vi "Arrays.vi"() -> ()   [LabVIEW 2018]
panel:
  out "Subset Array":dbl[][](array[numeric])
  out "Scaled Array":dbl[][](array[numeric])
  out "Random Array":dbl[][](array[numeric])
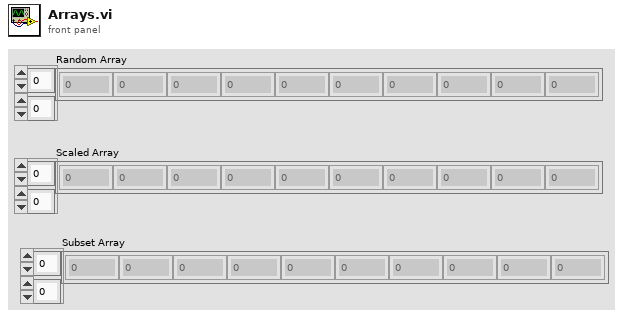
[diagram p1: front panel]
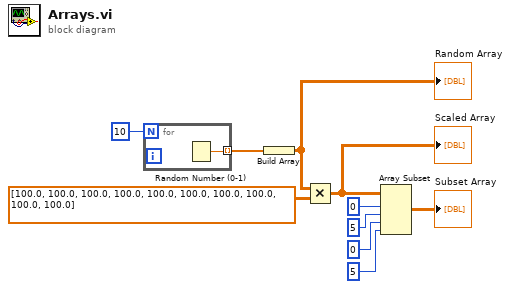
[diagram p0: block diagram]
diagram:
  n1 = for {
    N: 10 -> [_]
    tunnel: [w11] -> w10 mode=indexing
    n2 = Random Number (0-1)() -> (number: 0 to 1=w11:dbl)
  }
  n3 = Build Array(w10) -> (w8:dbl[][])
  "Random Array" <- w8
  n4 = Multiply(x=w8, y=dbl[][] [[100.0, 100.0, 100.0, 100.0, 100.0, 100.0, 100.0, 100.0, 100.0, 100.0]]) -> (x*y=w6:dbl[][])
  "Scaled Array" <- w6
  n5 = Array Subset(array=w6, index (row)=0 ("index"), length (row)=5 ("length"), index (col)=0 ("index"), length (col)=5 ("length")) -> (→"Subset Array":dbl[][])
